vi "dfd_Create CIC Filter.vi"(5 "mode":T2 items=["Default"=-1, "No Rate Change"=0, "Interpolation"=1, "Decimation"=2, "Interpolated"=3, "Rational"=4], 6 "fs in [Hz]":dbl=1.0, 7 "type":enum16{"Lowpass", "Highpass"}(ring), 8 "error in (no error)":errorcluster, 9 "lag":i32=1, 10 "factor":i32=1, 11 "num of stages":i32=2) -> (0 "error out":errorcluster, 3 "CIC filter out":T1={"mMRate_Structure"=enum."CIC", "mMRate_Mode"=0, "mMRate_Factor"=1, "mMRate_FIRParams"={"mMRate_FIR_H"=[], "mMRate_FIR_IsNyquist?"=FALSE, "mMRate_FIR_IsSymmetric?"=FALSE}, "mMRate_CICParams"={"mMRate_CIC_#Stage"=2, "mMRate_CIC_Lag"=1, "mMRate_CIC_Type"=enum."Lowpass"}, "mMRate_Order"=1, "mMRate_Version"="1.0", "mMRate_Comments"="1.0", "mMRate_RationalFactor"={"mMRate_L"=-1, "mMRate_M"=-1}, "mMRate_Fs"=1.0, "mMRate_Quantized?"=FALSE, "mMRate_QFilterGain"=1.0, "mMRate_CoefWl"=16, "mMRate_Scaling"={"mMRate_ScaleByPowerOf2?"=FALSE, "mMRate_ScaleType"=enum."Time Domain 1-Norm"}, "mMRate_InputWl"=0, "mMRate_OutputWl"=0, "mMRate_OutputMode"=enum."Nearest", "mMRate_MultMode"=enum."Truncated", "mMRate_BitPruning"=FALSE, "mMRate_GainWl"=16, "mMRate_OutputFwl"=0, "mMRate_SumIwl"=0, "mMRate_InputIwl "=16, "mMRate_SumWl"=32, "mMRate_CoefIwl"=0} {"mMRate_SumWl" min=1 max=32 step=1; "mMRate_InputIwl" min=1 max=32 step=1; "mMRate_GainWl" min=1 max=32 step=1; "mMRate_OutputWl" min=1 max=32 step=1; "mMRate_InputWl" min=1 max=32 step=1; "mMRate_CoefWl" min=1 max=32 step=1; "mMRate_Mode" items=["Default"=-1, "No Rate Change"=0, "Interpolation"=1, "Decimation"=2, "Interpolated"=3, "Rational"=4]})   [LabVIEW 2017, in "NI_DigFilterLicensed.lvlib"]
uses:
  <vilib>/addons/Digital Filter Design/NI_DigFilterLicensed.lvlib
  <vilib>/addons/Digital Filter Design/_Objects.llb/DFD Multirate Mode.ctl
  <vilib>/addons/Digital Filter Design/_Objects.llb/DFD Multirate Filter Obj.ctl
  <vilib>/addons/Digital Filter Design/_Objects.llb/DFD Coef Norm Type.ctl
  <vilib>/addons/Digital Filter Design/_Objects.llb/DFD Round-off Mode.ctl
  <vilib>/addons/Digital Filter Design/_Objects.llb/DFD FXP MRate Multiply Mode.ctl
  <vilib>/Analysis/2dsp.llb/1D Convolution (DBL).vi
  <vilib>/addons/Digital Filter Design/_Misc.llb/dfd_Error Handlers (Single).vi
  <vilib>/Analysis/NI_AALPro.lvlib
panel:
  in  "multirate filter":T1={"mMRate_Structure"=enum."IIR", "mMRate_Mode"=0, "mMRate_Factor"=-1, "mMRate_FIRParams"={"mMRate_FIR_H"=[], "mMRate_FIR_IsNyquist?"=FALSE, "mMRate_FIR_IsSymmetric?"=FALSE}, "mMRate_CICParams"={"mMRate_CIC_#Stage"=0, "mMRate_CIC_Lag"=0, "mMRate_CIC_Type"=enum."Lowpass"}, "mMRate_Order"=0, "mMRate_Version"="2.0", "mMRate_Comments"="", "mMRate_RationalFactor"={"mMRate_L"=-1, "mMRate_M"=-1}, "mMRate_Fs"=1.0, "mMRate_Quantized?"=FALSE, "mMRate_QFilterGain"=1.0, "mMRate_CoefWl"=16, "mMRate_Scaling"={"mMRate_ScaleByPowerOf2?"=FALSE, "mMRate_ScaleType"=enum."No Norm"}, "mMRate_InputWl"=16, "mMRate_OutputWl"=16, "mMRate_OutputMode"=enum."Truncation", "mMRate_MultMode"=enum."Truncated", "mMRate_BitPruning"=FALSE, "mMRate_GainWl"=16, "mMRate_OutputFwl"=0, "mMRate_SumIwl"=0, "mMRate_InputIwl "=16, "mMRate_SumWl"=32, "mMRate_CoefIwl"=0} {"mMRate_SumWl" min=1 max=32 step=1; "mMRate_InputIwl" min=1 max=32 step=1; "mMRate_GainWl" min=1 max=32 step=1; "mMRate_OutputWl" min=1 max=32 step=1; "mMRate_InputWl" min=1 max=32 step=1; "mMRate_CoefWl" min=1 max=32 step=1; "mMRate_Mode" items=["Default"=-1, "No Rate Change"=0, "Interpolation"=1, "Decimation"=2, "Interpolated"=3, "Rational"=4]}
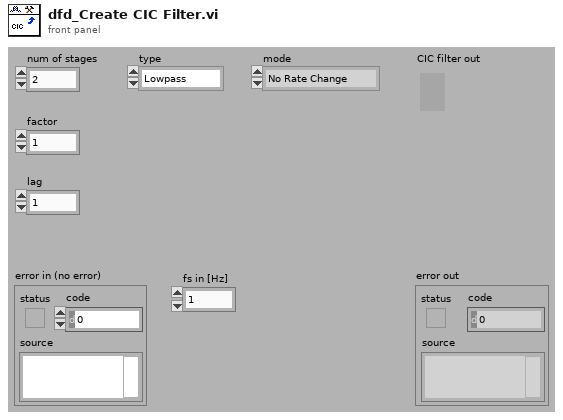
[diagram p1: front panel]
types:
  T1 = typedef "NI_DigFilterLicensed.lvlib/DFD Multirate Filter Obj.ctl" = cluster{"mMRate_Structure":enum16{"CIC", "FIR", "IIR", "Lattice"}, "mMRate_Mode":T2, "mMRate_Factor":i32, "mMRate_FIRParams":cluster{"mMRate_FIR_H":dbl[], "mMRate_FIR_IsNyquist?":bool, "mMRate_FIR_IsSymmetric?":bool}, "mMRate_CICParams":cluster{"mMRate_CIC_#Stage":i32, "mMRate_CIC_Lag":i32, "mMRate_CIC_Type":enum16{"Lowpass", "Highpass"}}, "mMRate_Order":i32, "mMRate_Version":string, "mMRate_Comments":string, "mMRate_RationalFactor":cluster{"mMRate_L":i32, "mMRate_M":i32}, "mMRate_Fs":dbl, "mMRate_Quantized?":bool, "mMRate_QFilterGain":dbl, "mMRate_CoefWl":i16, "mMRate_Scaling":cluster{"mMRate_ScaleByPowerOf2?":bool, "mMRate_ScaleType":T3}, "mMRate_InputWl":i16, "mMRate_OutputWl":i16, "mMRate_OutputMode":T4, "mMRate_MultMode":T5, "mMRate_BitPruning":bool, "mMRate_GainWl":i16, "mMRate_OutputFwl":i16, "mMRate_SumIwl":i16, "mMRate_InputIwl ":i16, "mMRate_SumWl":i16, "mMRate_CoefIwl":i16}
  T2 = typedef "NI_DigFilterLicensed.lvlib/DFD Multirate Mode.ctl" = i16
  T3 = typedef "NI_DigFilterLicensed.lvlib/DFD Coef Norm Type.ctl" = enum16{"No Norm", "Time Domain 1-Norm", "Time Domain 2-Norm", "Time Domain Inf-Norm"}
  T4 = typedef "NI_DigFilterLicensed.lvlib/DFD Round-off Mode.ctl" = enum16{"Nearest", "Truncation"}
  T5 = typedef "NI_DigFilterLicensed.lvlib/DFD FXP MRate Multiply Mode.ctl" = enum16{"Truncated", "Full"}
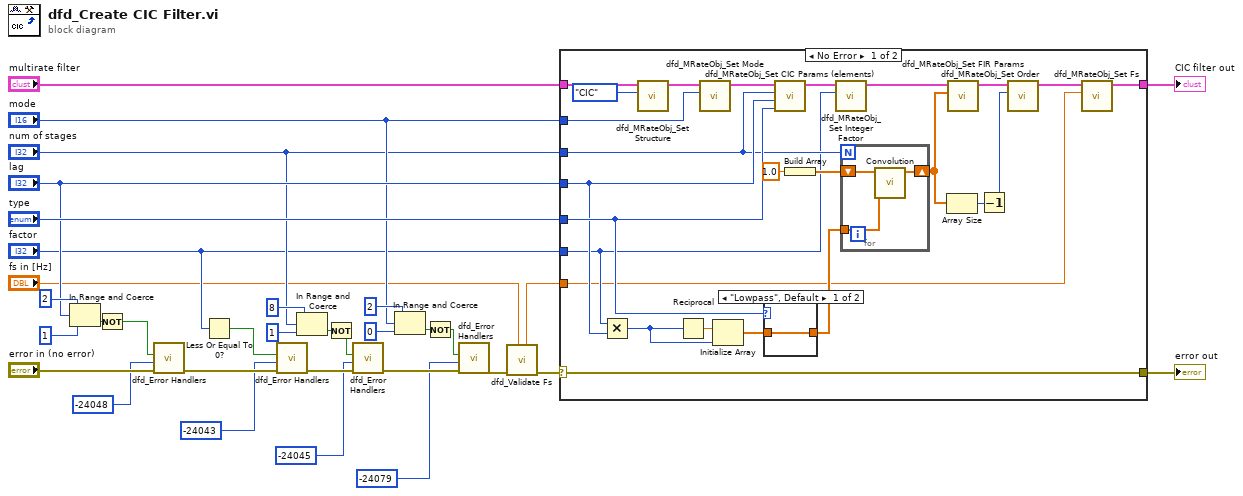
[diagram p0: block diagram]
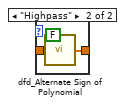
[diagram p2: hidden frame]
diagram:
  n1 = In Range and Coerce(upper limit=2, x="lag", lower limit=1) -> (In Range?=w20:bool)  [unwired: 1 out]
  n2 = Not(x=w20) -> (.not. x?=w19:bool)
  n3 = call-poly <vilib>:"dfd_Error Handlers.vi"("error in (no error)"="error in (no error)", "error code"=-24048 ("ERR_LAG_RANGE"), "condition failed?"=w19) -> ("error out"=w31:errorcluster)  [unwired: 8 out]
  n4 = Less Or Equal To 0?(x="factor") -> (x <= 0?=w6:bool)
  n5 = call-poly <vilib>:"dfd_Error Handlers.vi"("error in (no error)"=w31, "error code"=-24043 ("ERR_FACTOR_LE_ZERO"), "condition failed?"=w6) -> ("error out"=w29:errorcluster)  [unwired: 8 out]
  n6 = In Range and Coerce(upper limit=8, x="num of stages", lower limit=1) -> (In Range?=w11:bool)  [unwired: 1 out]
  n7 = Not(x=w11) -> (.not. x?=w7:bool)
  n8 = call-poly <vilib>:"dfd_Error Handlers.vi"("error in (no error)"=w29, "error code"=-24045 ("ERR_#STAGE_RANGE"), "condition failed?"=w7) -> ("error out"=w18:errorcluster)  [unwired: 8 out]
  n9 = In Range and Coerce(upper limit=2, x="mode", lower limit=0) -> (In Range?=w13:bool)  [unwired: 1 out]
  n10 = Not(x=w13) -> (.not. x?=w12:bool)
  n11 = call-poly <vilib>:"dfd_Error Handlers.vi"("error in (no error)"=w18, "error code"=-24079 ("ERR_FILTERING_MODE"), "condition failed?"=w12) -> ("error out"=w4:errorcluster)  [unwired: 8 out]
  n12 = call <vilib>:"dfd_Validate Fs.vi"("fs [Hz]"="fs in [Hz]", "error in (no error)"=w4) -> ("error out"=w3:errorcluster, "dup fs [Hz]"=w1:dbl)  [unwired: 8 in]
  n13 = case shown="No Error" w3 {
    selector: w3 -> [w58 w67]
    tunnel: "factor" -> [w40 _]
    tunnel: "lag" -> [w48 _]
    tunnel: "num of stages" -> [w41 _]
    tunnel: "type" -> [w49 _]
    tunnel: "mode" -> [w50 _]
    tunnel: "multirate filter" -> [w51 w66]
    tunnel: [w36 w66] -> w25
    tunnel: [w58 w67] -> w24
    tunnel: w1 -> [w34 _]
    frame No Error {
      n14 = Multiply(x=w40, y=w48) -> (x*y=w53:i32)
      n15 = call <vilib>:"dfd_MRateObj_Set Structure.vi"("structure"=enum16{"CIC", "FIR", "IIR", "Lattice"}."CIC", "multirate filter in"=w51) -> ("multirate filter out"=w39:T1)  [unwired: 9 out]
      n16 = Reciprocal(x=w53) -> (1/x=w54:dbl)
      n17 = call <vilib>:"dfd_MRateObj_Set Mode.vi"("mode"=w50, "multirate filter in"=w39) -> ("multirate filter out"=w38:T1)  [unwired: 9 out]
      n18 = Initialize Array(w54, w53) -> (w55:dbl[])
      n19 = case shown="\"Lowpass\", Default" w49 {
        tunnel: w55 -> [w59 w62]
        tunnel: [w59 w61] -> w52
        frame "Lowpass", Default {
        }
        frame "Highpass" {
          n20 = call <vilib>:"dfd_Alternate Sign of Polynomial.vi"("polynomial in"=w62, "even? (F)"=FALSE) -> ("polynomial out"=w61:dbl[])
        }
      }
      n21 = call <vilib>:"dfd_MRateObj_Set CIC Params (elements).vi"("type"=w49, "lag"=w48, "# stages"=w41, "multirate filter in"=w38) -> ("multirate filter out"=w37:T1)  [unwired: 7 out]
      n22 = Build Array(1.0 ("element")) -> (w57:dbl[])
      n23 = call <vilib>:"dfd_MRateObj_Set Integer Factor.vi"("factor"=w40, "multirate filter in"=w37) -> ("multirate filter out"=w47:T1)  [unwired: 9 out]
      n24 = for {
        N: w41 -> [_]
        tunnel: w52 -> [w64]
        shift-right: [w63] -> w44
        shift-left: w57 -> [w65]
        n25 = call-poly <vilib>:"Convolution.vi"("Y"=w64, "X"=w65) -> ("X * Y"=w63:dbl[])  [unwired: 1 in, 8 out]
      }
      n26 = Array Size(array=w44) -> (size(s)=w43:i32)
      n27 = call <vilib>:"dfd_MRateObj_Set FIR Params.vi"("h(n)"=w44, "multirate filter in"=w47) -> ("multirate filter out"=w46:T1)  [unwired: 2 in, 7 out]
      n28 = Decrement(x=w43) -> (x-1=w42:i32)
      n29 = call <vilib>:"dfd_MRateObj_Set Order.vi"("order"=w42, "multirate filter in"=w46) -> ("multirate filter out"=w45:T1)  [unwired: 9 out]
      n30 = call <vilib>:"dfd_MRateObj_Set Fs.vi"("fs"=w34, "multirate filter in"=w45) -> ("dup multirate filter"=w36:T1)  [unwired: 9 out]
    }
    frame Error {
    }
  }
  "error out" <- w24
  "CIC filter out" <- w25
